vi "Modra-Believer.vi"(11 "NXT/EV3":T1) -> (3 "NXT/EV3 2":T1)   [LabVIEW 2016]
uses:
  <vilib>/NXT/Subs/LVHSConnector.ctl
  <vilib>/NXT/LegoClasses/BrickReference/BrickReference.lvclass
  <vilib>/NXT/Dual Mode Library/Display/drawText_Center.vi
  <vilib>/NXT/Dual Mode Library/Sound/PlayA.vi
  <vilib>/NXT/Dual Mode Library/Sound/PlayE.vi
  <vilib>/NXT/Dual Mode Library/Sound/PlayD.vi
  <vilib>/NXT/Dual Mode Library/Sound/PlayC.vi
  <vilib>/NXT/Dual Mode Library/Sound/PlayG.vi
  <vilib>/NXT/Dual Mode Library/Waits/Wait_Num.vi
  <vilib>/NXT/Dual Mode Library/Sound/PlayGsharp.vi
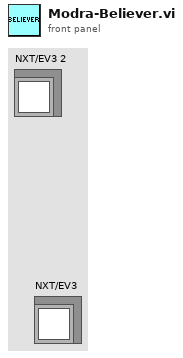
[diagram p1: front panel]
types:
  T1 = typedef "LVHSConnector.ctl" = refnum<class "BrickReference.lvclass">
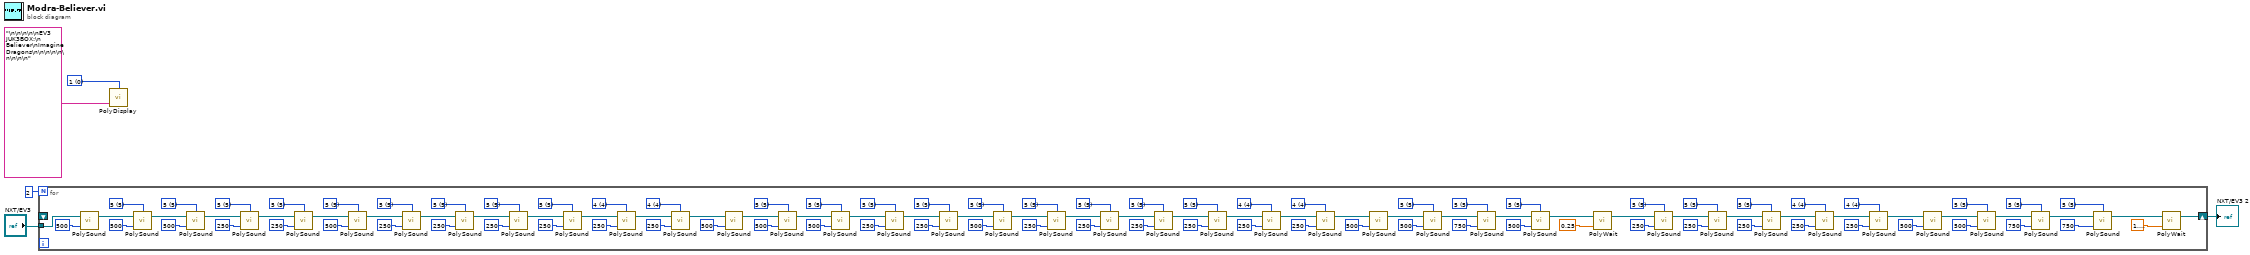
[diagram p0: block diagram]
diagram:
  w4 = i16 0 items=["1", "2", "3", "4", "5", "6", "7", "8", "9", "10", "11", "12"] ("Line")
  n1 = for {
    N: 2 -> [_]
    tunnel: "NXT/EV3" -> [w7]
    shift-right: [w6] -> w1
    shift-left: _ -> [_]
    w12 = u16 5 items=["3"=3, "4"=4, "5"=5, "6"=6, "7"=7] ("Octave")
    w19 = u16 5 items=["3"=3, "4"=4, "5"=5, "6"=6, "7"=7] ("Octave")
    w15 = u16 5 items=["3"=3, "4"=4, "5"=5, "6"=6, "7"=7] ("Octave")
    w30 = u16 4 items=["3"=3, "4"=4, "5"=5, "6"=6, "7"=7] ("Octave")
    w29 = u16 4 items=["3"=3, "4"=4, "5"=5, "6"=6, "7"=7] ("Octave")
    w26 = u16 5 items=["3"=3, "4"=4, "5"=5, "6"=6, "7"=7] ("Octave")
    w23 = u16 5 items=["3"=3, "4"=4, "5"=5, "6"=6, "7"=7] ("Octave")
    w21 = u16 5 items=["3"=3, "4"=4, "5"=5, "6"=6, "7"=7] ("Octave")
    w40 = u16 5 items=["3"=3, "4"=4, "5"=5, "6"=6, "7"=7] ("Octave")
    w42 = u16 5 items=["3"=3, "4"=4, "5"=5, "6"=6, "7"=7] ("Octave")
    w47 = u16 5 items=["3"=3, "4"=4, "5"=5, "6"=6, "7"=7] ("Octave")
    w80 = u16 4 items=["3"=3, "4"=4, "5"=5, "6"=6, "7"=7] ("Octave")
    w79 = u16 4 items=["3"=3, "4"=4, "5"=5, "6"=6, "7"=7] ("Octave")
    w76 = u16 5 items=["3"=3, "4"=4, "5"=5, "6"=6, "7"=7] ("Octave")
    w72 = u16 5 items=["3"=3, "4"=4, "5"=5, "6"=6, "7"=7] ("Octave")
    w68 = u16 5 items=["3"=3, "4"=4, "5"=5, "6"=6, "7"=7] ("Octave")
    w69 = u16 5 items=["3"=3, "4"=4, "5"=5, "6"=6, "7"=7] ("Octave")
    w64 = u16 5 items=["3"=3, "4"=4, "5"=5, "6"=6, "7"=7] ("Octave")
    w59 = u16 5 items=["3"=3, "4"=4, "5"=5, "6"=6, "7"=7] ("Octave")
    w58 = u16 5 items=["3"=3, "4"=4, "5"=5, "6"=6, "7"=7] ("Octave")
    w54 = u16 5 items=["3"=3, "4"=4, "5"=5, "6"=6, "7"=7] ("Octave")
    w52 = u16 5 items=["3"=3, "4"=4, "5"=5, "6"=6, "7"=7] ("Octave")
    w87 = u16 4 items=["3"=3, "4"=4, "5"=5, "6"=6, "7"=7] ("Octave")
    w88 = u16 4 items=["3"=3, "4"=4, "5"=5, "6"=6, "7"=7] ("Octave")
    w91 = u16 5 items=["3"=3, "4"=4, "5"=5, "6"=6, "7"=7] ("Octave")
    w95 = u16 5 items=["3"=3, "4"=4, "5"=5, "6"=6, "7"=7] ("Octave")
    w99 = u16 5 items=["3"=3, "4"=4, "5"=5, "6"=6, "7"=7] ("Octave")
    w98 = u16 5 items=["3"=3, "4"=4, "5"=5, "6"=6, "7"=7] ("Octave")
    w103 = u16 5 items=["3"=3, "4"=4, "5"=5, "6"=6, "7"=7] ("Octave")
    w108 = u16 5 items=["3"=3, "4"=4, "5"=5, "6"=6, "7"=7] ("Octave")
    w109 = u16 5 items=["3"=3, "4"=4, "5"=5, "6"=6, "7"=7] ("Octave")
    w113 = u16 5 items=["3"=3, "4"=4, "5"=5, "6"=6, "7"=7] ("Octave")
    w115 = u16 5 items=["3"=3, "4"=4, "5"=5, "6"=6, "7"=7] ("Octave")
    n2 = call-poly <vilib>:"PolySound.vi"("Duration (500 ms)"=u16 500, "NXT/EV3"=w7) -> ("NXT/EV3"=w114:T1)  [unwired: 2 in]
    n3 = call-poly <vilib>:"PolySound.vi"("Duration (500 ms)"=u16 500, "NXT/EV3"=w114, "Octave"=w115) -> ("NXT/EV3"=w111:T1)  [unwired: 1 in]
    n4 = call-poly <vilib>:"PolySound.vi"("Duration (500 ms)"=u16 500, "NXT/EV3"=w111, "Octave"=w113) -> ("NXT/EV3"=w105:T1)  [unwired: 1 in]
    n5 = call-poly <vilib>:"PolySound.vi"("Duration (500 ms)"=u16 250, "NXT/EV3"=w105, "Octave"=w109) -> ("NXT/EV3"=w106:T1)  [unwired: 1 in]
    n6 = call-poly <vilib>:"PolySound.vi"("Duration (500 ms)"=u16 250, "NXT/EV3"=w106, "Octave"=w108) -> ("NXT/EV3"=w102:T1)  [unwired: 1 in]
    n7 = call-poly <vilib>:"PolySound.vi"("Duration (500 ms)"=u16 500, "NXT/EV3"=w102, "Octave"=w103) -> ("NXT/EV3"=w96:T1)  [unwired: 1 in]
    n8 = call-poly <vilib>:"PolySound.vi"("Duration (500 ms)"=u16 250, "NXT/EV3"=w96, "Octave"=w98) -> ("NXT/EV3"=w101:T1)  [unwired: 1 in]
    n9 = call-poly <vilib>:"PolySound.vi"("Duration (500 ms)"=u16 250, "NXT/EV3"=w101, "Octave"=w99) -> ("NXT/EV3"=w93:T1)  [unwired: 1 in]
    n10 = call-poly <vilib>:"PolySound.vi"("Duration (500 ms)"=u16 250, "NXT/EV3"=w93, "Octave"=w95) -> ("NXT/EV3"=w90:T1)  [unwired: 1 in]
    n11 = call-poly <vilib>:"PolySound.vi"("Duration (500 ms)"=u16 250, "NXT/EV3"=w90, "Octave"=w91) -> ("NXT/EV3"=w85:T1)  [unwired: 1 in]
    n12 = call-poly <vilib>:"PolySound.vi"("Duration (500 ms)"=u16 250, "NXT/EV3"=w85, "Octave"=w88) -> ("NXT/EV3"=w84:T1)  [unwired: 1 in]
    n13 = call-poly <vilib>:"PolySound.vi"("Duration (500 ms)"=u16 250, "NXT/EV3"=w84, "Octave"=w87) -> ("NXT/EV3"=w49:T1)  [unwired: 1 in]
    n14 = call-poly <vilib>:"PolySound.vi"("Duration (500 ms)"=u16 500, "NXT/EV3"=w49) -> ("NXT/EV3"=w53:T1)  [unwired: 2 in]
    n15 = call-poly <vilib>:"PolySound.vi"("Duration (500 ms)"=u16 500, "NXT/EV3"=w53, "Octave"=w52) -> ("NXT/EV3"=w56:T1)  [unwired: 1 in]
    n16 = call-poly <vilib>:"PolySound.vi"("Duration (500 ms)"=u16 500, "NXT/EV3"=w56, "Octave"=w54) -> ("NXT/EV3"=w62:T1)  [unwired: 1 in]
    n17 = call-poly <vilib>:"PolySound.vi"("Duration (500 ms)"=u16 250, "NXT/EV3"=w62, "Octave"=w58) -> ("NXT/EV3"=w61:T1)  [unwired: 1 in]
    n18 = call-poly <vilib>:"PolySound.vi"("Duration (500 ms)"=u16 250, "NXT/EV3"=w61, "Octave"=w59) -> ("NXT/EV3"=w65:T1)  [unwired: 1 in]
    n19 = call-poly <vilib>:"PolySound.vi"("Duration (500 ms)"=u16 500, "NXT/EV3"=w65, "Octave"=w64) -> ("NXT/EV3"=w71:T1)  [unwired: 1 in]
    n20 = call-poly <vilib>:"PolySound.vi"("Duration (500 ms)"=u16 250, "NXT/EV3"=w71, "Octave"=w69) -> ("NXT/EV3"=w66:T1)  [unwired: 1 in]
    n21 = call-poly <vilib>:"PolySound.vi"("Duration (500 ms)"=u16 250, "NXT/EV3"=w66, "Octave"=w68) -> ("NXT/EV3"=w74:T1)  [unwired: 1 in]
    n22 = call-poly <vilib>:"PolySound.vi"("Duration (500 ms)"=u16 250, "NXT/EV3"=w74, "Octave"=w72) -> ("NXT/EV3"=w77:T1)  [unwired: 1 in]
    n23 = call-poly <vilib>:"PolySound.vi"("Duration (500 ms)"=u16 250, "NXT/EV3"=w77, "Octave"=w76) -> ("NXT/EV3"=w82:T1)  [unwired: 1 in]
    n24 = call-poly <vilib>:"PolySound.vi"("Duration (500 ms)"=u16 250, "NXT/EV3"=w82, "Octave"=w79) -> ("NXT/EV3"=w83:T1)  [unwired: 1 in]
    n25 = call-poly <vilib>:"PolySound.vi"("Duration (500 ms)"=u16 250, "NXT/EV3"=w83, "Octave"=w80) -> ("NXT/EV3"=w44:T1)  [unwired: 1 in]
    n26 = call-poly <vilib>:"PolySound.vi"("Duration (500 ms)"=u16 500, "NXT/EV3"=w44) -> ("NXT/EV3"=w48:T1)  [unwired: 2 in]
    n27 = call-poly <vilib>:"PolySound.vi"("Duration (500 ms)"=u16 500, "NXT/EV3"=w48, "Octave"=w47) -> ("NXT/EV3"=w41:T1)  [unwired: 1 in]
    n28 = call-poly <vilib>:"PolySound.vi"("Duration (500 ms)"=u16 750, "NXT/EV3"=w41, "Octave"=w42) -> ("NXT/EV3"=w38:T1)  [unwired: 1 in]
    n29 = call-poly <vilib>:"PolySound.vi"("Duration (500 ms)"=u16 500, "NXT/EV3"=w38, "Octave"=w40) -> ("NXT/EV3"=w37:T1)  [unwired: 1 in]
    n30 = call-poly <vilib>:"PolyWait.vi"("Time (1 sec)"=sgl 0.25, "NXT/EV3"=w37) -> ("NXT/EV3"=w34:T1)  [unwired: 2 in]
    n31 = call-poly <vilib>:"PolySound.vi"("Duration (500 ms)"=u16 250, "NXT/EV3"=w34, "Octave"=w21) -> ("NXT/EV3"=w22:T1)  [unwired: 1 in]
    n32 = call-poly <vilib>:"PolySound.vi"("Duration (500 ms)"=u16 250, "NXT/EV3"=w22, "Octave"=w23) -> ("NXT/EV3"=w27:T1)  [unwired: 1 in]
    n33 = call-poly <vilib>:"PolySound.vi"("Duration (500 ms)"=u16 250, "NXT/EV3"=w27, "Octave"=w26) -> ("NXT/EV3"=w32:T1)  [unwired: 1 in]
    n34 = call-poly <vilib>:"PolySound.vi"("Duration (500 ms)"=u16 250, "NXT/EV3"=w32, "Octave"=w29) -> ("NXT/EV3"=w33:T1)  [unwired: 1 in]
    n35 = call-poly <vilib>:"PolySound.vi"("Duration (500 ms)"=u16 250, "NXT/EV3"=w33, "Octave"=w30) -> ("NXT/EV3"=w13:T1)  [unwired: 1 in]
    n36 = call-poly <vilib>:"PolySound.vi"("Duration (500 ms)"=u16 500, "NXT/EV3"=w13) -> ("NXT/EV3"=w14:T1)  [unwired: 2 in]
    n37 = call-poly <vilib>:"PolySound.vi"("Duration (500 ms)"=u16 500, "NXT/EV3"=w14, "Octave"=w15) -> ("NXT/EV3"=w20:T1)  [unwired: 1 in]
    n38 = call-poly <vilib>:"PolySound.vi"("Duration (500 ms)"=u16 750, "NXT/EV3"=w20, "Octave"=w19) -> ("NXT/EV3"=w10:T1)  [unwired: 1 in]
    n39 = call-poly <vilib>:"PolySound.vi"("Duration (500 ms)"=u16 750, "NXT/EV3"=w10, "Octave"=w12) -> ("NXT/EV3"=w8:T1)  [unwired: 1 in]
    n40 = call-poly <vilib>:"PolyWait.vi"("Time (1 sec)"=sgl 1.4, "NXT/EV3"=w8) -> ("NXT/EV3"=w6:T1)  [unwired: 2 in]
  }
  "NXT/EV3 2" <- w1
  n41 = call-poly <vilib>:"PolyDisplay.vi"("Text"="\n\n\n\n\nEV3 JUK3BOX:\n Believer\nImagine Dragons\n\n\n\n\n\n\n\n\n", "Line"=w4) -> ()  [unwired: 2 in, 1 out]
